vi "Launch Application.vi"() -> ()   [LabVIEW 2014]
uses:
  <vilib>/ActorFramework/Actor/Actor.lvclass
  Controller/TEC Controller.lvclass
panel:
  out "error out":errorcluster
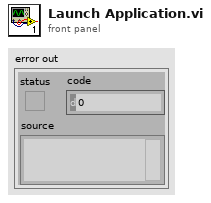
[diagram p1: front panel]
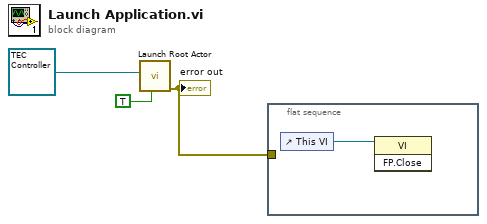
[diagram p0: block diagram]
diagram:
  n1 = call <vilib>:"Launch Root Actor.vi"("Open Actor Core front panel? (F)"=TRUE, "Actor"=refnum<class "TEC Controller.lvclass"> refnum ("Humidifier Test Lib.lvlib:TEC Controller")) -> ("error out"=w1:errorcluster)  [unwired: 8 in, 1 out]
  "error out" <- w1
  n2 = flat-sequence {
    tunnel: w1 -> [_]
    frame #0 {
      n3 = control-ref of="This VI"() -> (w4:refnum<vi>)
      n4 = invoke class="VI" method="FP.Close"(reference=w4) -> ()  [unwired: 2 in, 3 out]
    }
  }
